vi "AdquisicioDadesRadiacio.vi"(8 "Stop":refnum<vi>, 10 "EventDades":refnum<user-event>, 11 "AssaigActiu":refnum<vi>) -> (0 "error out":errorcluster)   [LabVIEW 2017]
uses:
  <vilib>/DAQmx/read.llb/DAQmx Read (Analog 1D DBL 1Chan NSamp).vi
  <vilib>/DAQmx/miscellaneous.llb/DAQmx Fill In Error Info.vi
  <resource>/objmgr/daqmx.rc
panel:
  out "IncT":dbl
  out "SampClk.Rate":dbl
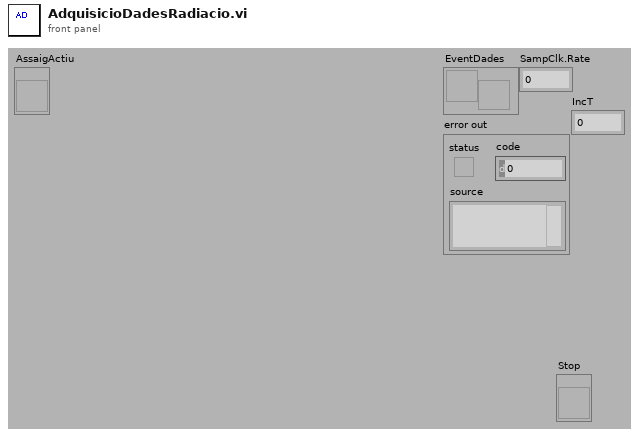
[diagram p1: front panel]
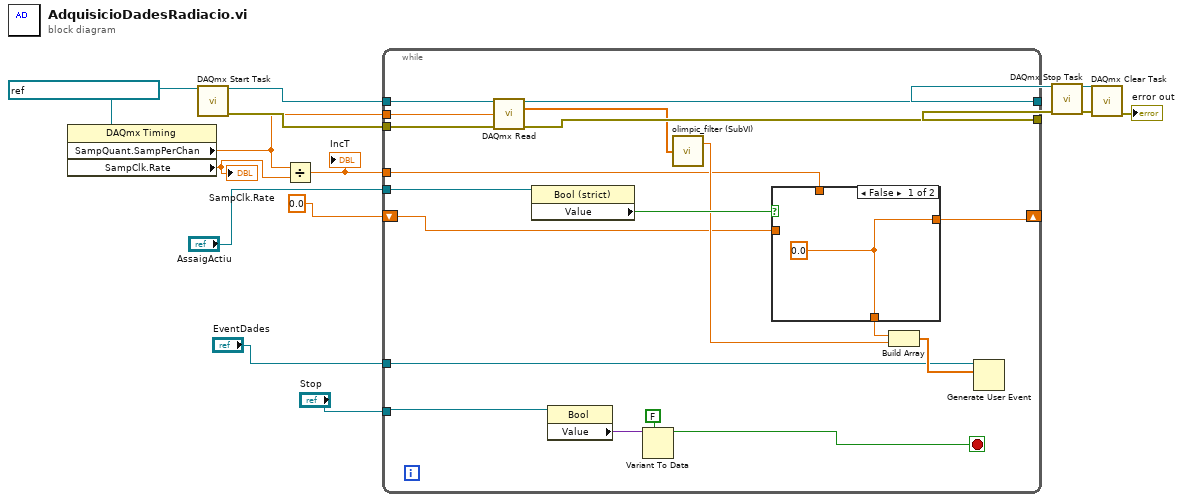
[diagram p0: block diagram]
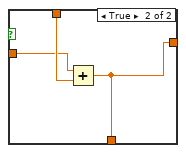
[diagram p2: hidden frame]
diagram:
  w8 = refnum<k21> "USB_Equip_Radiacio_T1" ("task/channels in")
  n1 = property class="DAQmx Timing"(reference=w8) -> ("SampQuant.SampPerChan"=w3:dbl, "SampClk.Rate"=w2:dbl)  [unwired: 1 in, 2 out]
  "SampClk.Rate" <- w2
  n2 = call <vilib>:"DAQmx Start Task.vi"("task/channels in"=w8) -> ("task out"=w14:refnum<k21>, "error out"=w13:errorcluster)  [unwired: 13 in]
  n3 = Divide(x=w3, y=w2) -> (x/y=w1:dbl)
  "IncT" <- w1
  n4 = while {
    tunnel: w14 -> [w27]
    tunnel: [w28] -> w15
    tunnel: w13 -> [w34]
    tunnel: "Stop" -> [w33]
    tunnel: [w30] -> w11
    shift-right: [w21] -> _
    shift-left: 0.0 ("relative seconds") -> [w22]
    tunnel: "EventDades" -> [w19]
    tunnel: "AssaigActiu" -> [w18]
    tunnel: w3 -> [w17]
    tunnel: w1 -> [w16]
    stop <- w29 stop-if-true
    n5 = call-poly <vilib>:"DAQmx Read.vi"("task/channels in"=w27, "number of samples per channel"=w17, "error in"=w34) -> ("task out"=w28:refnum<k21>, "data"=w26:dbl[], "error out"=w30:errorcluster)  [unwired: 10 in]
    n6 = property class="Bool (strict)"(reference=w18) -> ("Value"=w25:bool)  [unwired: 1 in, 2 out]
    n7 = property class="Bool"(reference=w33) -> ("Value"=w32:variant)  [unwired: 1 in, 2 out]
    n8 = Variant To Data(type=FALSE, Variant=w32) -> (data=w29:bool)  [unwired: 1 in, 1 out]
    n9 = call "olimpic_filter (SubVI).vi"("array"=w26) -> ("olimpic_filter"=w23:sgl)  [unwired: 1 out]
    n10 = case shown="False" w25 {
      tunnel: w22 -> [_ w37]
      tunnel: [w35 w36] -> w24
      tunnel: [w35 w36] -> w21
      tunnel: w16 -> [_ w38]
      frame False {
        w35 = 0.0
      }
      frame True {
        n11 = Add(x=w37, y=w38) -> (x+y=w36:dbl)
      }
    }
    n12 = Build Array(w24, w23) -> (w20:dbl[])
    n13 = Generate User Event(user event=w19, event data cluster=w20) -> ()  [unwired: 2 in, 2 out]
  }
  n14 = call <vilib>:"DAQmx Stop Task.vi"("task/channels in"=w15, "error in"=w11) -> ("task out"=w10:refnum<k21>, "error out"=w9:errorcluster)  [unwired: 12 in]
  n15 = call <vilib>:"DAQmx Clear Task.vi"("task in"=w10, "error in"=w9) -> ("error out"=→"error out":errorcluster)  [unwired: 13 in]
